vi "test_se_main.vi"() -> ()   [LabVIEW 2016]
uses:
  <vilib>/rvi/DesktopExecutionNode/Execution/niFpgaDEN_Execute.vi
  <vilib>/rvi/DesktopExecutionNode/DesktopExecutionNode.xnode
panel:
  out "Array":T1(array[cluster])
  out "debug":T2(array[cluster])
  in  "se.p.fastBlanking":T3
  in  "se.mot.p.target":cluster{"x":fxp<+/-,16,1>, "y":fxp<+/-,16,1>}[](array[cluster])
  in  "scanTurnOnTime":i32[](array[numeric])
  in  "outputParams":T4={"se.p.scanOffsets"={"x"=0.0, "y"=0.0}, "se.p.transformMatrix"={"a"=1.0, "b"=0.0, "c"=0.0, "d"=1.0}, "se.p.scanSize"={"fastScanSize"=0.0, "slowScanSize"=0.0, "invertSlowAxis"=FALSE}}
  out "clocks":T5(array[cluster])
  in  "se.p.modes":T6
  in  "se.mot.p.clocks":T7={"moveToDecFactor"=9, "moveToWaveSize"=128, "se.mot.p.invDec"=0.0}
  in  "se.p.clocks":T8={"outputRate"=50, "fastDecFactor"=4, "outWaveSizeFast"=128, "pplUpsampling"=4, "numLines"=16, "se.p.fastInvDec"=0.0, "se.p.slowUpStep"=0.0, "se.p.outWaveSizeSlow"=128, "blankingMax"=0}
  out "simulationProgressDone":dbl(slide) scale=0.0..1.0
  out "XY Graph":cluster{i32[], i16[]}[](graph)
  out "output":T9(array[cluster])
  in  "simulationTime (ticks)":i32
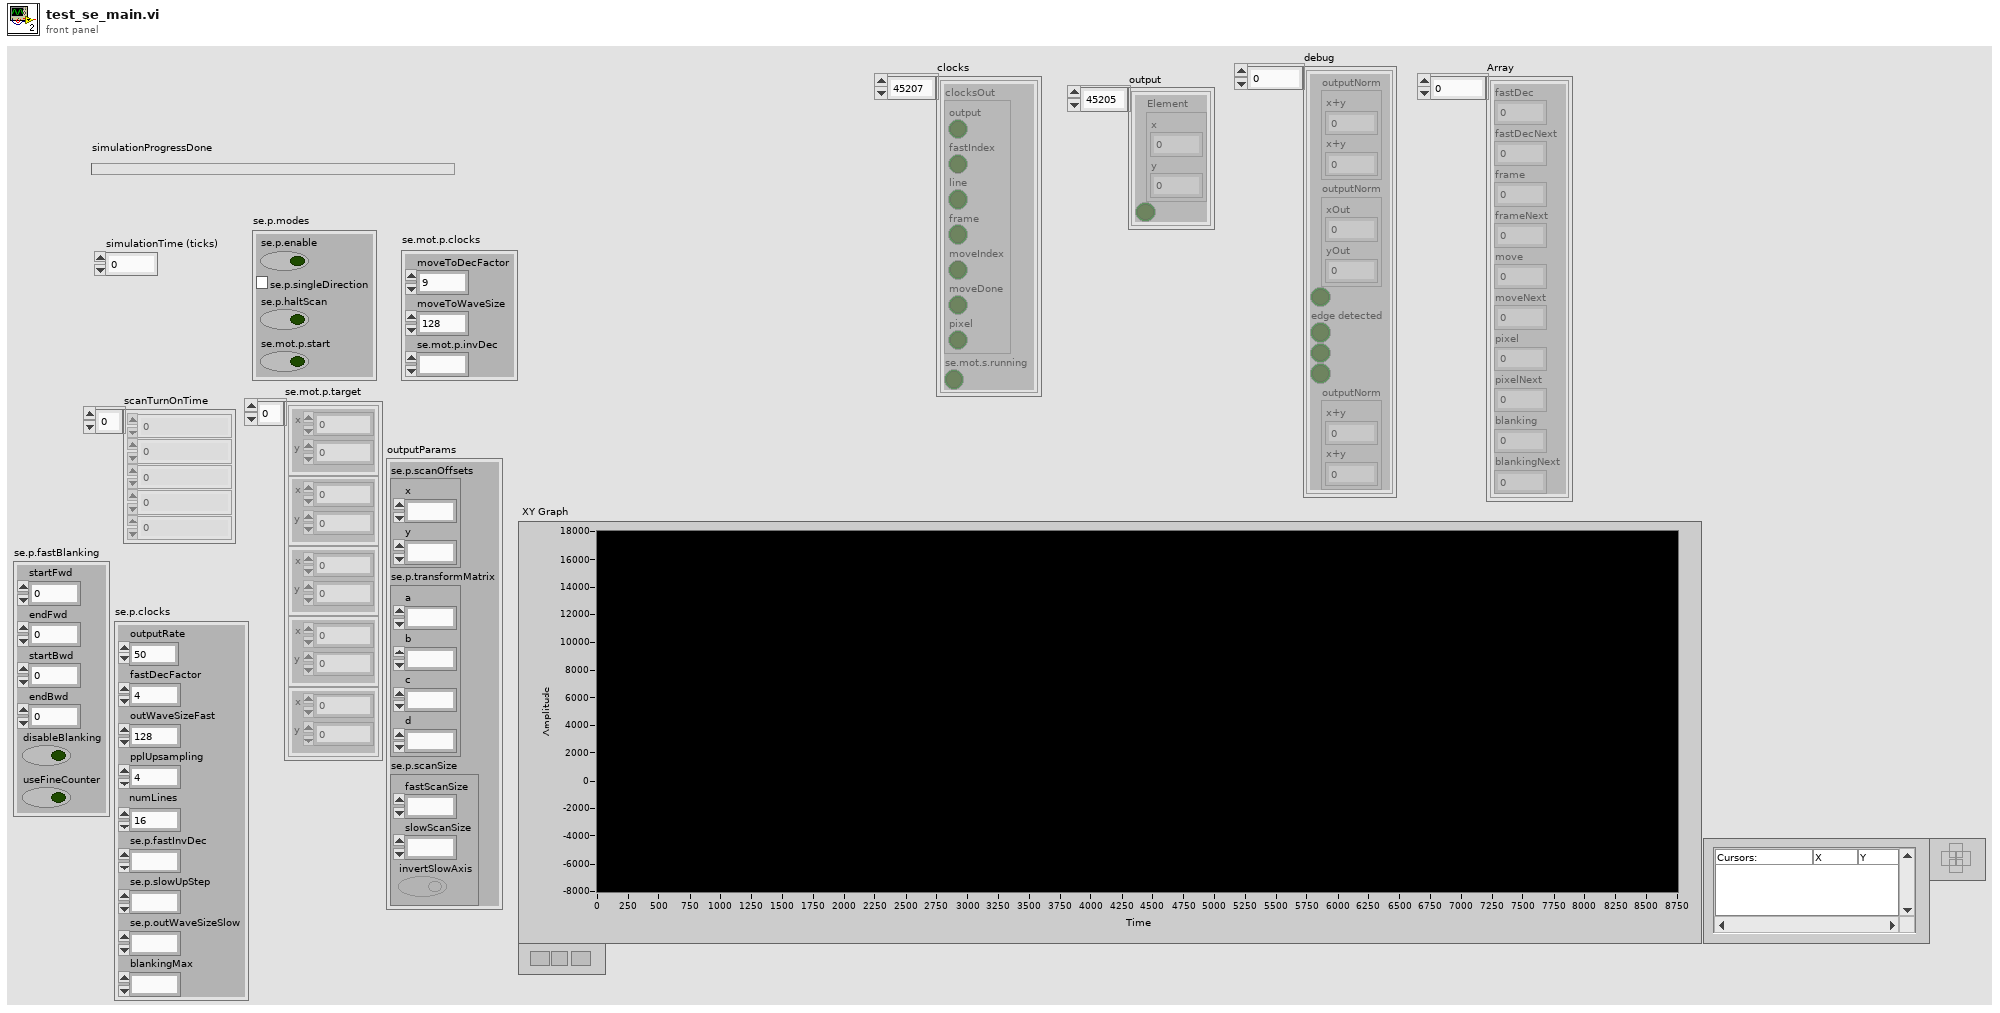
[diagram p1: front panel]
types:
  T1 = cluster{"fastDec":u16, "fastDecNext":u16, "frame":u16, "frameNext":u16, "move":u16, "moveNext":u16, "pixel":u16, "pixelNext":u16, "blanking":u32, "blankingNext":u32}[]
  T2 = cluster{"outputNorm":cluster{"x+y":fxp<+/-,18,2>, "x+y":fxp<+/-,18,2>}, "outputNorm":cluster{"xOut":fxp<+/-,18,2>, "yOut":fxp<+/-,18,2>}, bool, "edge detected":bool, bool, bool, "outputNorm":cluster{"x+y":fxp<+/-,18,2>, "x+y":fxp<+/-,18,2>}}[]
  T3 = cluster{"startFwd":u32, "endFwd":u32, "startBwd":u32, "endBwd":u32, "disableBlanking":bool, "useFineCounter":bool}
  T4 = cluster{"se.p.scanOffsets":cluster{"x":fxp<+/-,16,1>, "y":fxp<+/-,16,1>}, "se.p.transformMatrix":cluster{"a":fxp<+/-,18,2>, "b":fxp<+/-,18,2>, "c":fxp<+/-,18,2>, "d":fxp<+/-,18,2>}, "se.p.scanSize":cluster{"fastScanSize":fxp<+,17,1>, "slowScanSize":fxp<+,17,1>, "invertSlowAxis":bool}}
  T5 = cluster{"clocksOut":cluster{"output":bool, "fastIndex":bool, "line":bool, "frame":bool, "moveIndex":bool, "moveDone":bool, "pixel":bool}, "se.mot.s.running":bool}[]
  T6 = cluster{"se.p.enable":bool, "se.p.singleDirection":bool, "se.p.haltScan":bool, "se.mot.p.start":bool}
  T7 = cluster{"moveToDecFactor":u16, "moveToWaveSize":u16, "se.mot.p.invDec":fxp<+,16,0>}
  T8 = cluster{"outputRate":u16, "fastDecFactor":u16, "outWaveSizeFast":u16, "pplUpsampling":u16, "numLines":u16, "se.p.fastInvDec":fxp<+,22,0>, "se.p.slowUpStep":fxp<+,22,0>, "se.p.outWaveSizeSlow":u16, "blankingMax":u32}
  T9 = cluster{"Element":cluster{"x":i16, "y":i16}, bool}[]
  T10 = cluster{"se.mot.p.clocks":cluster{"moveToDecFactor":u16, "moveToWaveSize":u16, "se.mot.p.invDec":fxp<+,16,0>}, "se.p.clocks":cluster{"outputRate":u16, "fastDecFactor":u16, "outWaveSizeFast":u16, "pplUpsampling":u16, "numLines":u16, "se.p.fastInvDec":fxp<+,22,0>, "se.p.slowUpStep":fxp<+,22,0>, "se.p.outWaveSizeSlow":u16, "blankingMax":u32}}
  T11 = cluster{"output":bool, "fastIndex":bool, "line":bool, "frame":bool, "moveIndex":bool, "moveDone":bool, "pixel":bool}
  T12 = cluster{"x+y":fxp<+/-,18,2>, "x+y":fxp<+/-,18,2>}
  T13 = cluster{"outputInt":cluster{"x":i16, "y":i16}, bool}
  T14 = cluster{"outputNorm":cluster{"x+y":fxp<+/-,18,2>, "x+y":fxp<+/-,18,2>}, "outputNorm":cluster{"xOut":fxp<+/-,18,2>, "yOut":fxp<+/-,18,2>}, bool, "edge detected":bool, bool, bool, "outputNorm":cluster{"x+y":fxp<+/-,18,2>, "x+y":fxp<+/-,18,2>}}
  T15 = cluster{"fastDec":u16, "fastDecNext":u16, "frame":u16, "frameNext":u16, "move":u16, "moveNext":u16, "pixel":u16, "pixelNext":u16, "blanking":u32, "blankingNext":u32}
  T16 = cluster{"clocksOut":cluster{"output":bool, "fastIndex":bool, "line":bool, "frame":bool, "moveIndex":bool, "moveDone":bool, "pixel":bool}, "se.mot.s.running":bool}
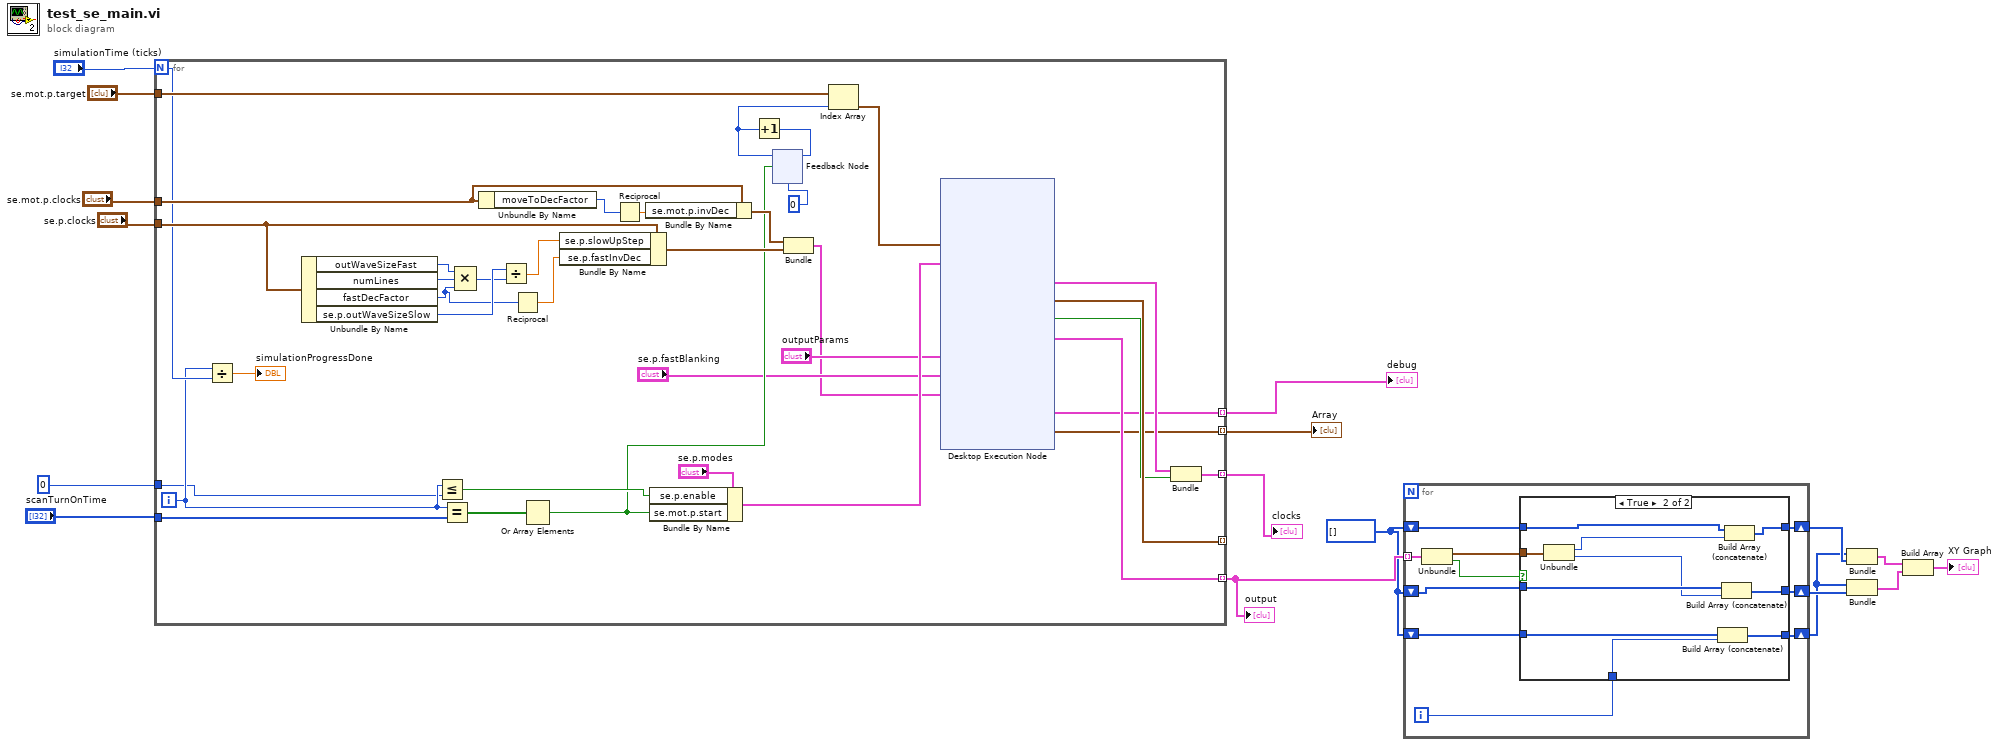
[diagram p0: block diagram]
diagram:
  w9 = i16[] []
  n1 = for {
    N: "simulationTime (ticks)" -> [w28]
    tunnel: [w53] -> w16 mode=indexing
    tunnel: [w52] -> _ mode=indexing
    tunnel: [w37] -> w8 mode=indexing
    tunnel: "se.mot.p.clocks" -> [w36]
    tunnel: "se.p.clocks" -> [w35]
    tunnel: "scanTurnOnTime" -> [w34]
    tunnel: "se.mot.p.target" -> [w30]
    tunnel: 0 -> [w26]
    tunnel: [w20] -> w2 mode=indexing
    tunnel: [w19] -> w1 mode=indexing
    i -> [w27]
    n2 = Divide(x=w27, y=w28) -> (x/y=→"simulationProgressDone":dbl)
    n3 = Unbundle By Name(w35) -> ("outWaveSizeFast"=w45:u16, "numLines"=w46:u16, "fastDecFactor"=w41:u16, "se.p.outWaveSizeSlow"=w44:u16)
    n4 = Less Or Equal?(x=w27, y=w26) -> (x <= y?=w29:bool)
    n5 = Equal?(x=w27, y=w34) -> (x = y?=w32:bool[])
    n6 = Compound Arithmetic op=MULTIPLY(w45, w46, w41) -> (w43:u16)
    n7 = Unbundle By Name(w36) -> ("moveToDecFactor"=w49:u16)
    n8 = Divide(x=w44, y=w43) -> (x/y=w42:dbl)
    n9 = Reciprocal(x=w41) -> (1/x=w40:dbl)
    n10 = Or Array Elements(Boolean array=w32) -> (logical OR=w25:bool)
    n11 = Bundle By Name(cluster=w35, "se.p.slowUpStep"=w42, "se.p.fastInvDec"=w40) -> (w51:T8)
    n12 = Reciprocal(x=w49) -> (1/x=w48:dbl)
    n13 = Bundle By Name(cluster=w36, "se.mot.p.invDec"=w48) -> (w50:T7)
    n14 = Bundle By Name(cluster="se.p.modes", "se.p.enable"=w29, "se.mot.p.start"=w25) -> (w47:T6)
    n15 = feedback #1(0) -> (w23:i32)
    n16 = Increment(x=w23) -> (x+1=w22:i32)
    n17 = feedback-in #1(w22, w25) -> ()
    n18 = Bundle("se.mot.p.clocks"=w50, "se.p.clocks"=w51) -> (w18:T10)  [unwired: 1 in]
    n19 = Index Array(array=w30, index=w23) -> (element=w31:cluster{"x":fxp<+/-,16,1>, "y":fxp<+/-,16,1>})
    n20 = xnode "Desktop Execution Node"("se.mot.p.target"=w31, "se.p.modes"=w47, "outputParams"="outputParams", "se.p.fastBlanking"="se.p.fastBlanking", "scanClocks"=w18) -> ("clocksOut"=w39:T11, "outputNorm"=w52:T12, "se.mot.s.running"=w38:bool, "se.o.position"=w53:T13, "debug"=w20:T14, "indices"=w19:T15)  [unwired: 1 in, 1 out]
    n21 = Bundle("clocksOut"=w39, "se.mot.s.running"=w38) -> (w37:T16)  [unwired: 1 in]
  }
  "output" <- w16
  "clocks" <- w8
  "debug" <- w2
  "Array" <- w1
  n22 = for {
    tunnel: w16 -> [w65] mode=indexing
    shift-right: [w63] -> w15
    shift-left: w9 -> [w64]
    shift-right: [w58] -> w14
    shift-left: w9 -> [w59]
    shift-right: [w57] -> w13
    shift-left: w9 -> [w56]
    i -> [w60]
    n23 = Unbundle(w65) -> ("outputInt"=w61:cluster{"x":i16, "y":i16}, w62:bool)
    n24 = case shown="True" w62 {
      tunnel: w64 -> [w68 w77]
      tunnel: [w68 w76] -> w63
      tunnel: w61 -> [_ w78]
      tunnel: w60 -> [_ w71]
      tunnel: w59 -> [w66 w75]
      tunnel: [w66 w74] -> w58
      tunnel: [w67 w70] -> w57
      tunnel: w56 -> [w67 w69]
      frame False {
      }
      frame True {
        n25 = Unbundle(w78) -> ("x"=w73:i16, "y"=w72:i16)
        n26 = Build Array (concatenate)(w69, w71) -> (w70:i32[])
        n27 = Build Array (concatenate)(w75, w72) -> (w74:i16[])
        n28 = Build Array (concatenate)(w77, w73) -> (w76:i16[])
      }
    }
  }
  n29 = Bundle(w13, w15) -> (w12:cluster{i32[], i16[]})  [unwired: 1 in]
  n30 = Bundle(w13, w14) -> (w10:cluster{i32[], i16[]})  [unwired: 1 in]
  n31 = Build Array(w12, w10) -> (→"XY Graph":cluster{i32[], i16[]}[])
